vi "LED_colors.vi"(9 "state":enum16{"Default", "Error", "No Error"}(ring)=enum."Error") -> (1 "Colors [4]":cluster{u32, u32}[](array[cluster]))   [LabVIEW 2015]
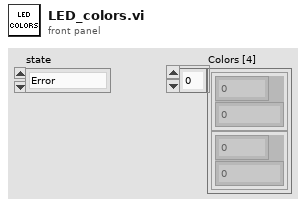
[diagram p1: front panel]
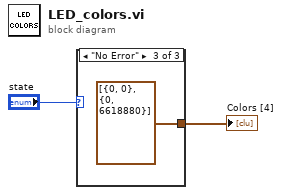
[diagram p0: block diagram]
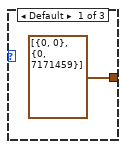
[diagram p2: hidden frame]
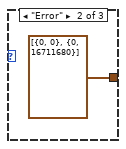
[diagram p3: hidden frame]
diagram:
  n1 = case shown="\"No Error\"" "state" {
    tunnel: [cluster{u32, u32}[] [{0, 0}, {0, 7171459}] ("Colors [4]") cluster{u32, u32}[] [{0, 0}, {0, 16711680}] ("Colors [4]") cluster{u32, u32}[] [{0, 0}, {0, 6618880}] ("Colors [4]")] -> w1
    frame Default {
    }
    frame "Error" {
    }
    frame "No Error" {
    }
  }
  "Colors [4]" <- w1
